vi "ConfigSetterTemplate.vi"(6 "timeoutSeconds":dbl, 8 "error in":errorcluster, 9 "FutureProofConfigs":bool, 10 "Configs":string, 11 "DeviceReference":T1) -> (0 "error out":errorcluster)   [LabVIEW 2023]
uses:
  <vilib>/Rock Robotics/WPI/ThirdParty/Phoenix6/DeviceReference.ctl
panel:
  out "StatusCode":i32
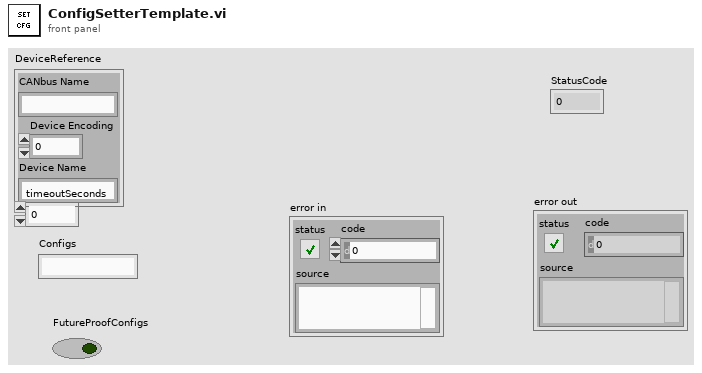
[diagram p1: front panel]
types:
  T1 = typedef "DeviceReference.ctl" = cluster{"CANbus Name":string, "Device Encoding":u32, "Device Name":string}
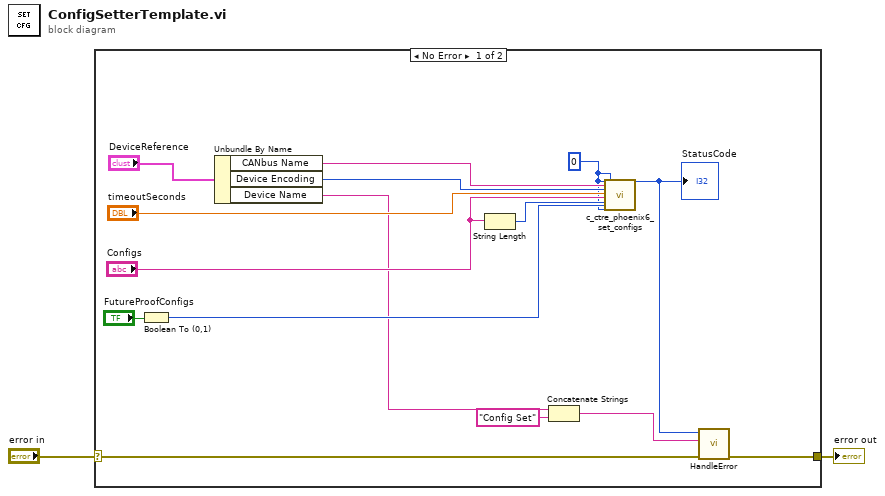
[diagram p0: block diagram]
diagram:
  n1 = case shown="No Error" "error in" {
    selector: "error in" -> [w7 w18]
    tunnel: [w6 w18] -> w1
    frame No Error {
      w9 = 0 ("Numeric 2")
      n2 = Boolean To (0,1)(Boolean="FutureProofConfigs") -> (0, 1=w10:i16)
      n3 = Unbundle By Name("DeviceReference") -> ("CANbus Name"=w16:string, "Device Encoding"=w15:u32, "Device Name"=w5:string)
      n4 = String Length(string="Configs") -> (length=w12:i32)
      n5 = Concatenate Strings(w5, "Config Set" ("string")) -> (w3:string)
      n6 = call <vilib>:"c_ctre_phoenix6_set_configs.vi"("Numeric 2"=w9, "String 2"=w16, "Numeric 3"=w15, "Numeric 4"="timeoutSeconds", "String 4"="Configs", "Numeric 5"=w12, "Numeric 6"=w10, "Numeric 7"=w9, "Numeric 8"=w9) -> ("Numeric"=w8:i32)  [unwired: 16 in, 2 out]
      "StatusCode" <- w8
      n7 = call "HandleError.vi"("error in"=w7, "origin"=w3, "Status"=w8) -> ("error out"=w6:errorcluster)  [unwired: 8 in]
    }
    frame Error {
    }
  }
  "error out" <- w1
